vi "MB_TCP_7018.vi"(5 "Status Reference":T1, 6 "N":i32, 7 "Data Reference":T2, 9 "timeouts":T3={"conn_timeout"=1000, "reconn_timeout"=3000, "N attempt max"=3, "t_reset_TTL"=120000, "write_timeout"=10, "read_timeout"=500, "period"=100} {"t_reset_TTL" min=10 max=240000 step=1; "period" min=10 max=100000 step=1; "read_timeout" min=10 max=60000 step=1; "write_timeout" min=1 max=60000 step=1; "N attempt max" min=1 max=5 step=1; "reconn_timeout" min=10 max=240000 step=1; "conn_timeout" min=10 max=240000}, 10 "write enable":bool=TRUE, 11 "stop":bool) -> (0 "error out":errorcluster, 2 "errors":i32, 3 "Z3":u32)   [LabVIEW 2019, in "MB_TCP1.lvlib"]
uses:
  MB_TCP1.lvlib
  Timer Delay/Timers.lvlib
  NI_modbus_upd/NI_modbus_upd.lvlib
  NI_modbus_upd/MB Modbus Command.ctl
  ICPCON Registers/ICPCON Registers.lvlib
  ICPCON Status/ICPCON Status.lvlib
  Timer Delay/unix time 1ms.vi
  NI_modbus_upd/TCP/TCP.lvclass
  ICPCON Registers/Ctl/ICPCON Data.ctl
  ICPCON Status/Ctl/ICPCON Status.ctl
panel:
  out "stopped":bool
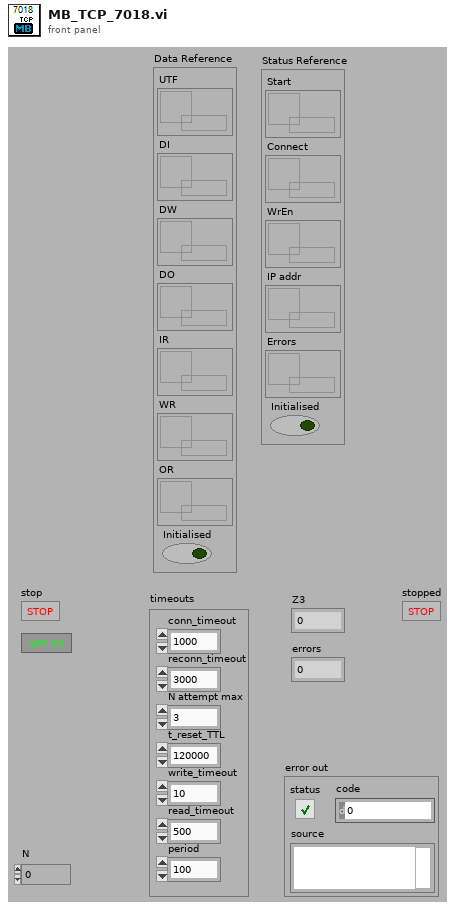
[diagram p1: front panel]
types:
  T1 = typedef "ICPCON Status.lvlib/ICPCON Status.ctl" = cluster{"Start":refnum<data-value>, "Connect":refnum<data-value>, "WrEn":refnum<data-value>, "IP addr":refnum<data-value>, "Errors":refnum<data-value>, "Initialised":bool}
  T2 = typedef "ICPCON Registers.lvlib/ICPCON Data.ctl" = cluster{"UTF":refnum<data-value>, "DI":refnum<data-value>, "DW":refnum<data-value>, "DO":refnum<data-value>, "IR":refnum<data-value>, "WR":refnum<data-value>, "OR":refnum<data-value>, "Initialised":bool}
  T3 = cluster{"conn_timeout":i32, "reconn_timeout":i32, "N attempt max":i32, "t_reset_TTL":i32, "write_timeout":i32, "read_timeout":i32, "period":i32}
  T4 = cluster{"Transaction ID":u16, "Protocol ID":u16, "Length":u16, "Unit ID":u8}
  T5 = typedef "NI_modbus_upd.lvlib/MB Modbus Command.ctl" = cluster{"Function Code":u8, "Starting Address":u16, "Quantity":u16, "Data":u16[], "Discrete":bool[]}
  T6 = cluster{"Remote IP Address":string, "Remote Port":u16}
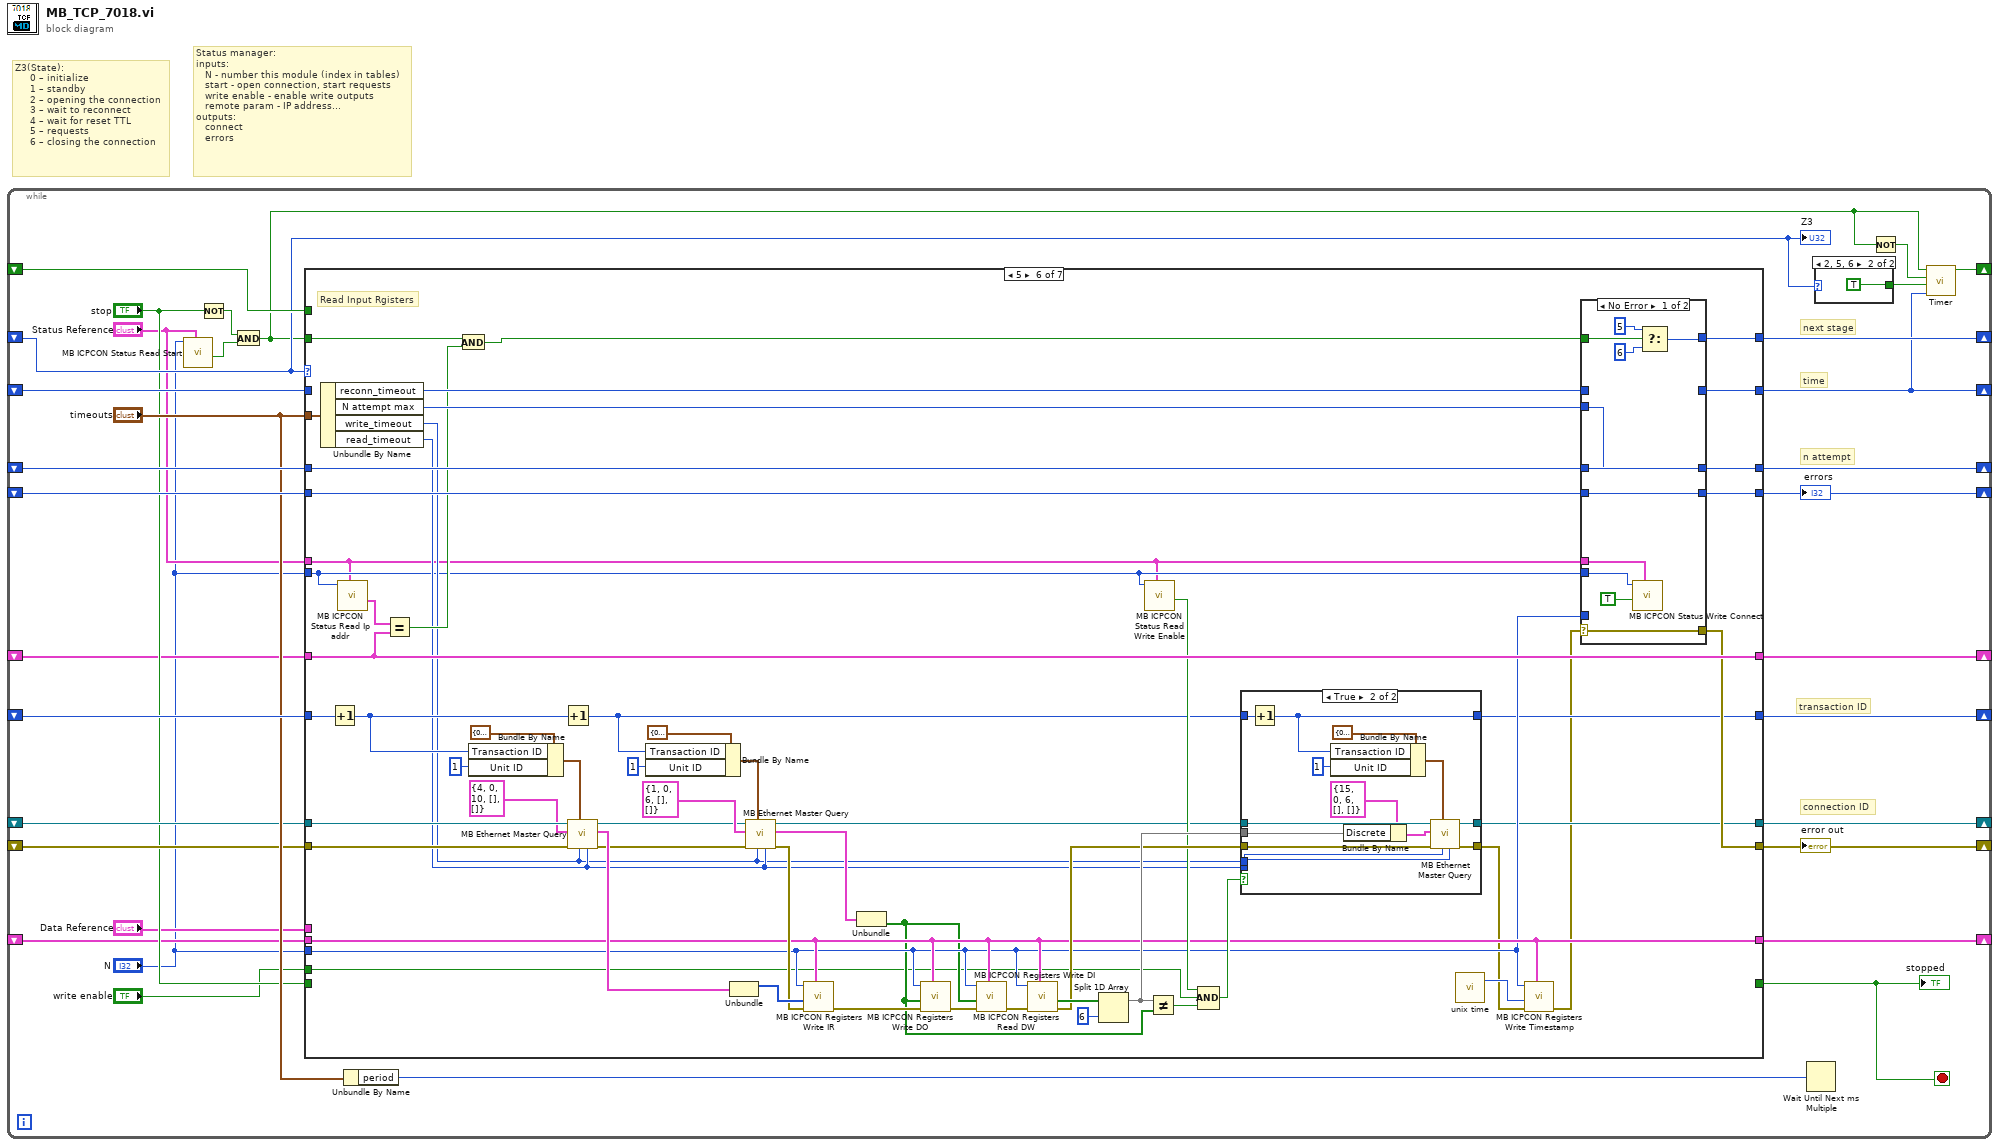
[diagram p0: block diagram]
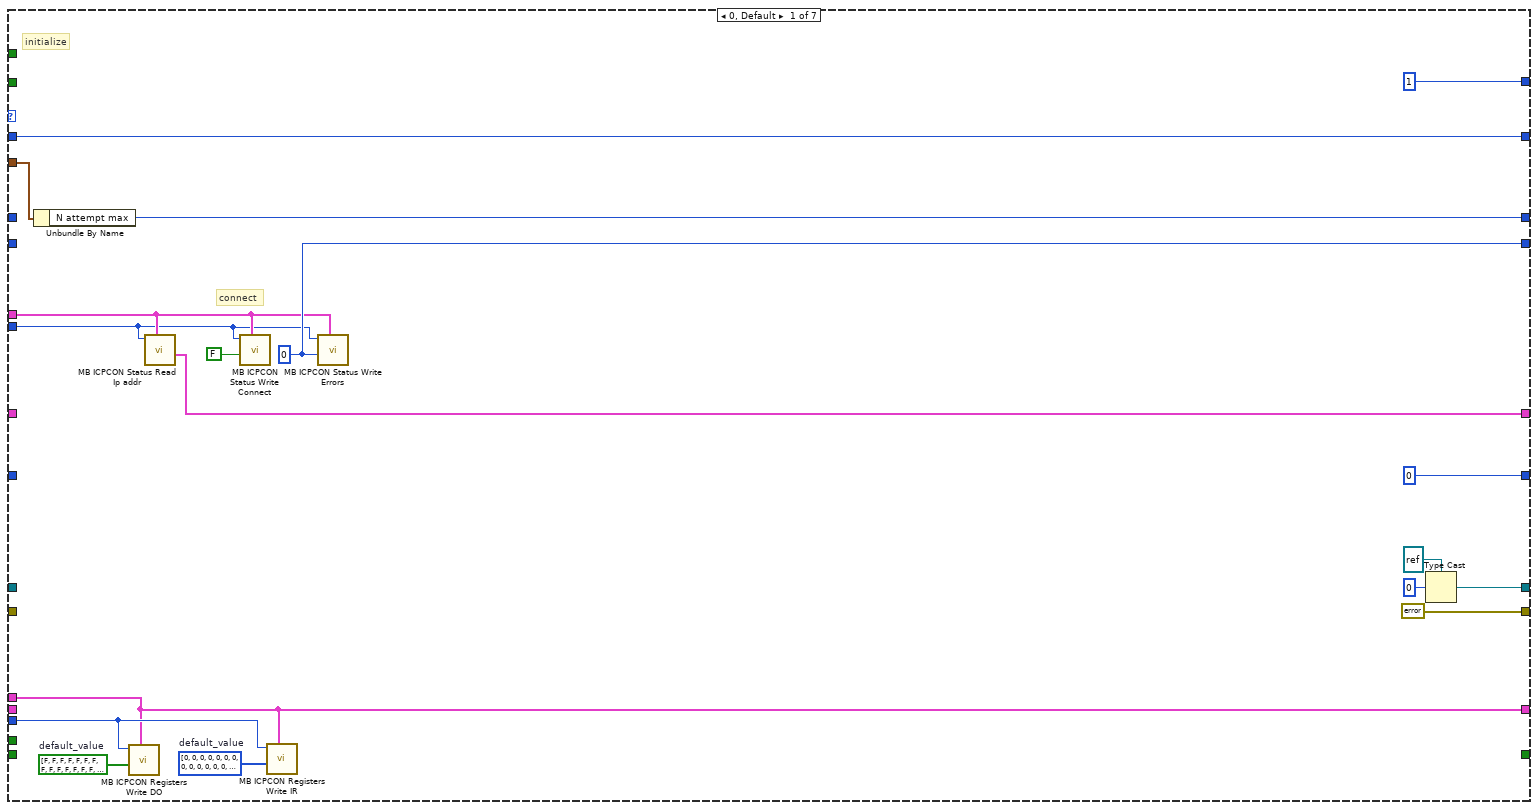
[diagram p2: hidden frame]
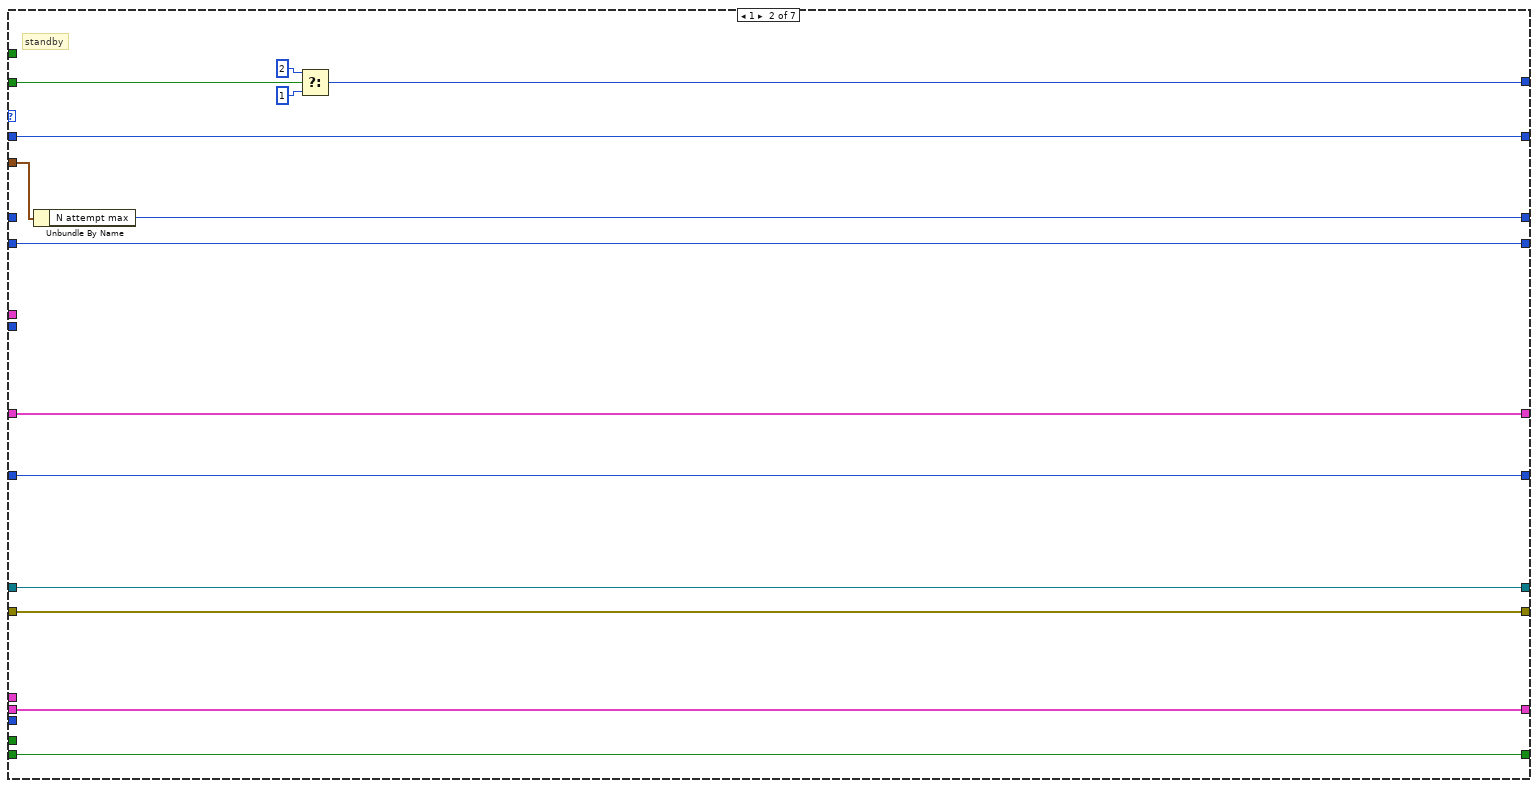
[diagram p3: hidden frame]
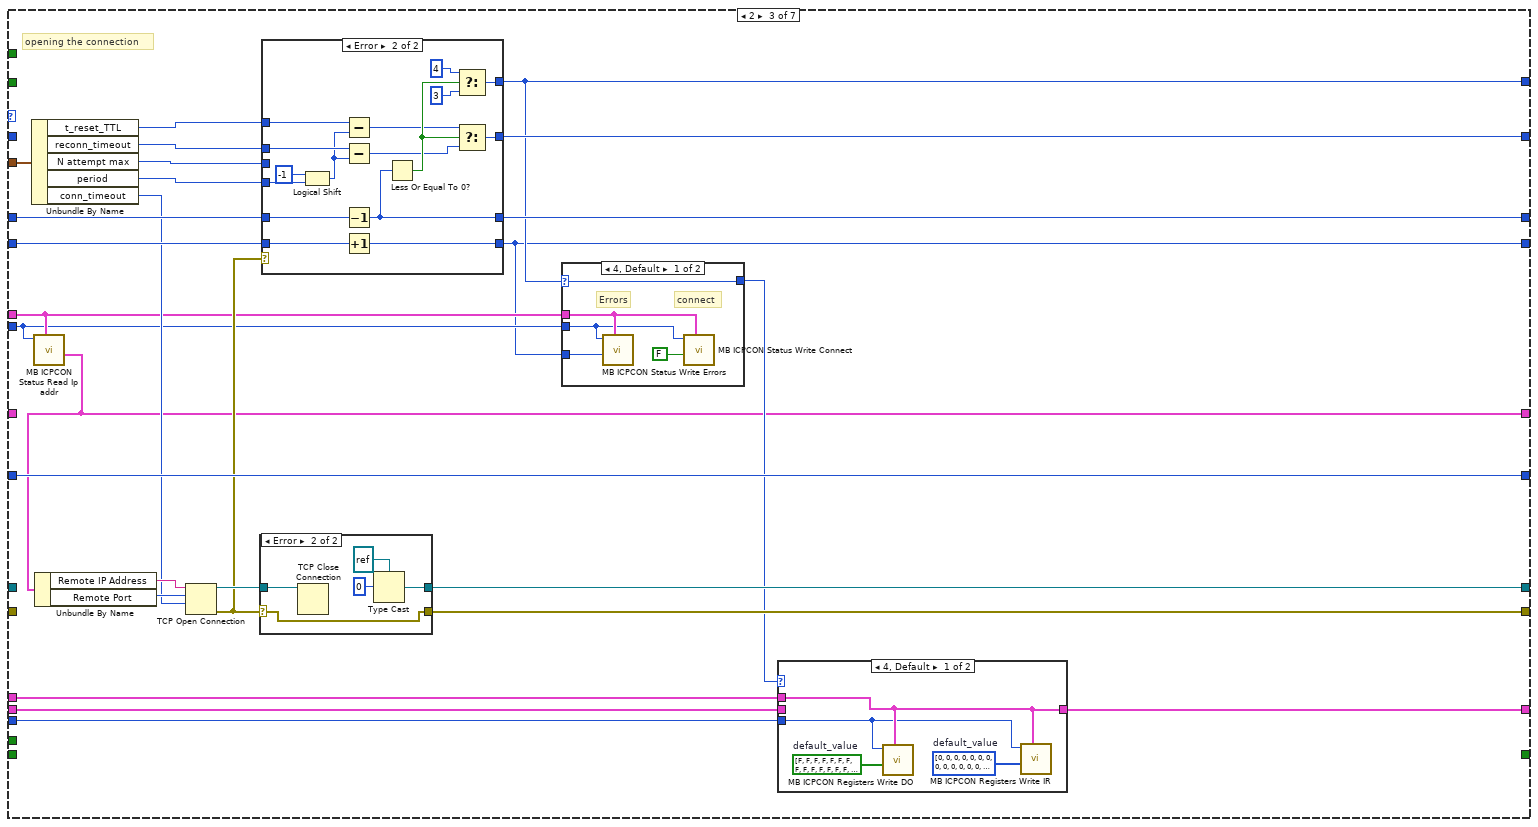
[diagram p4: hidden frame]
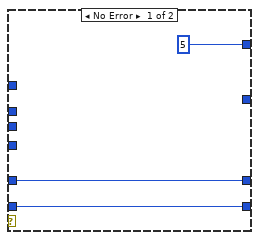
[diagram p8: hidden frame]
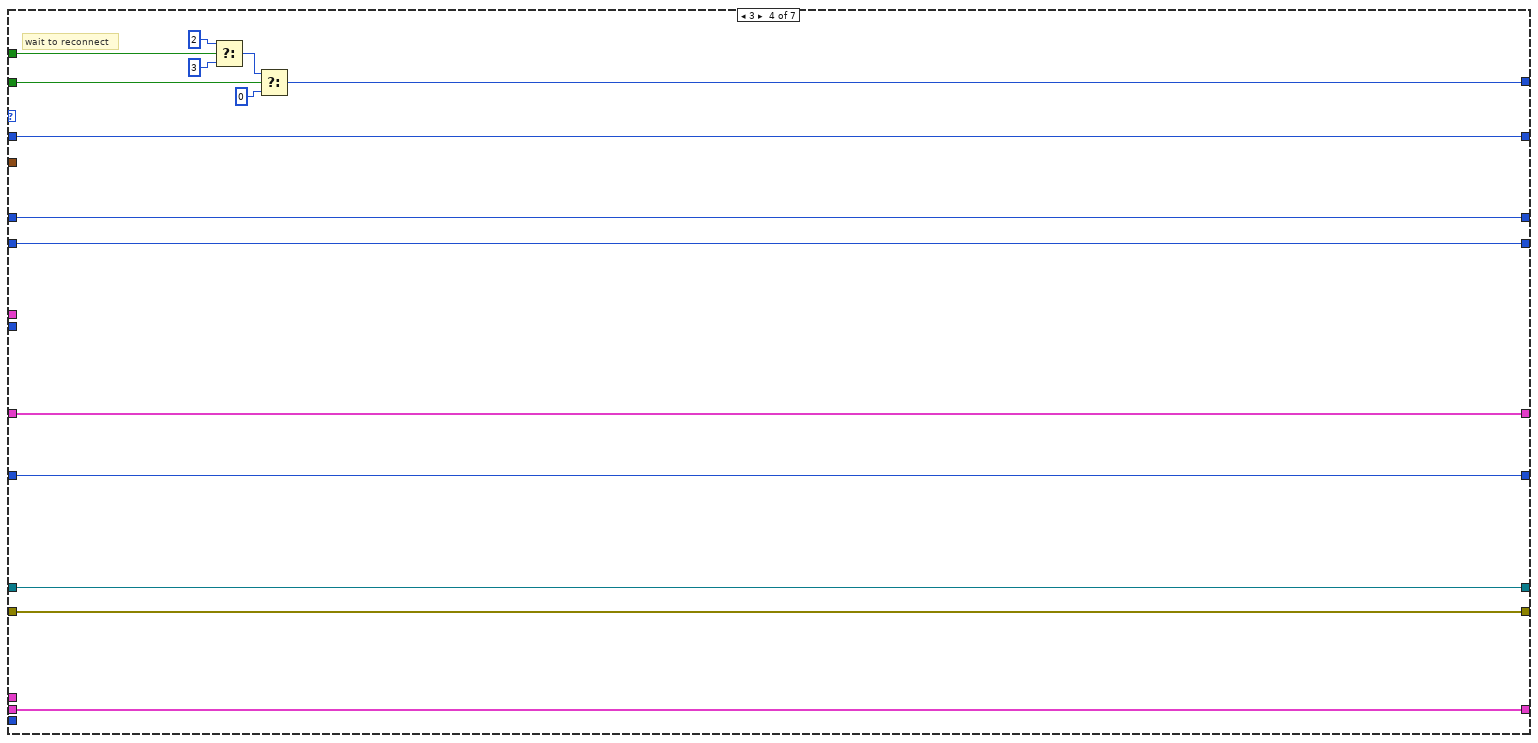
[diagram p9: hidden frame]
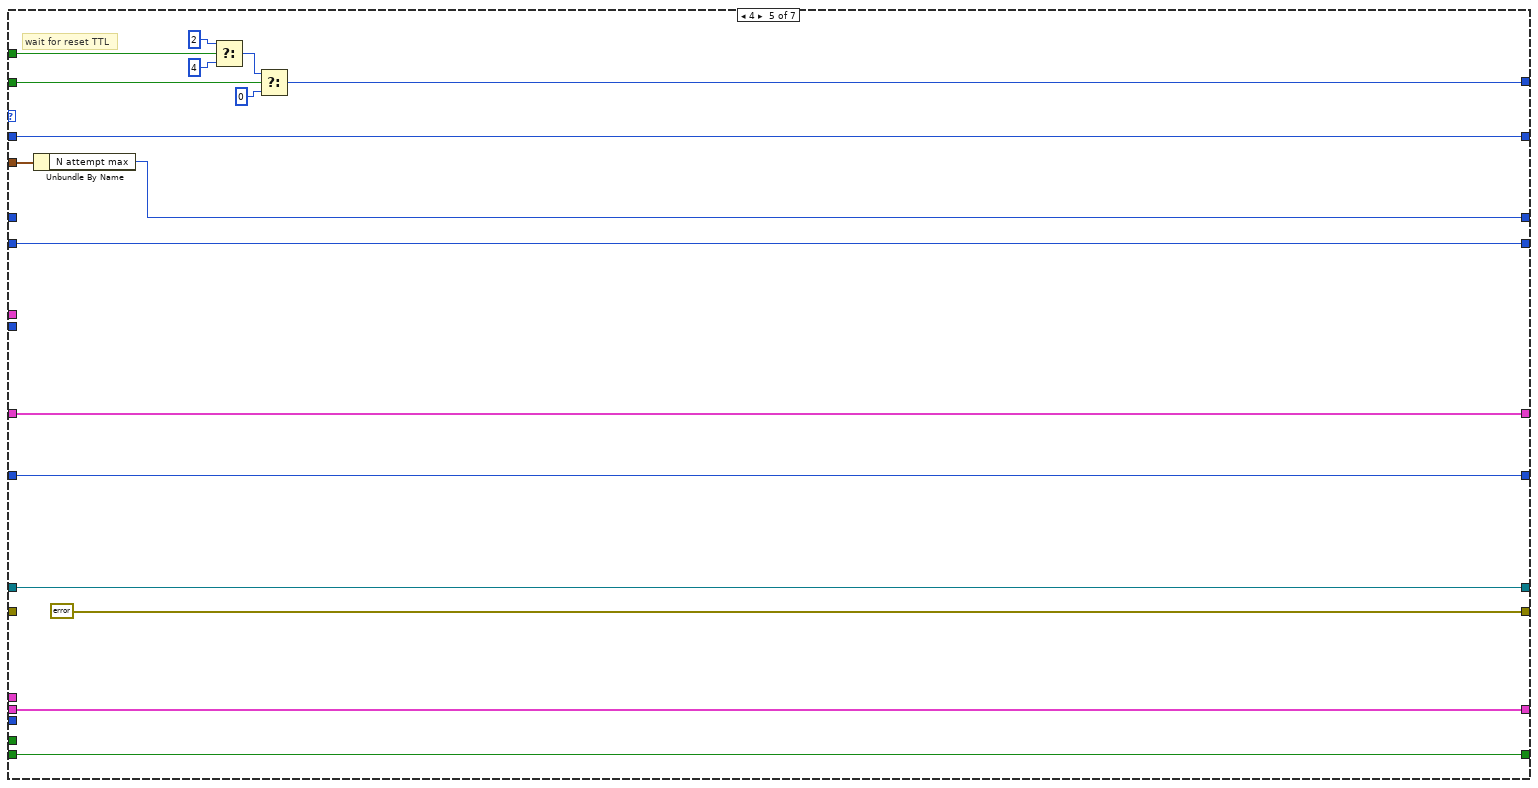
[diagram p10: hidden frame]
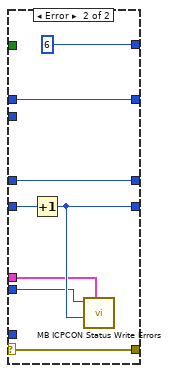
[diagram p12: hidden frame]
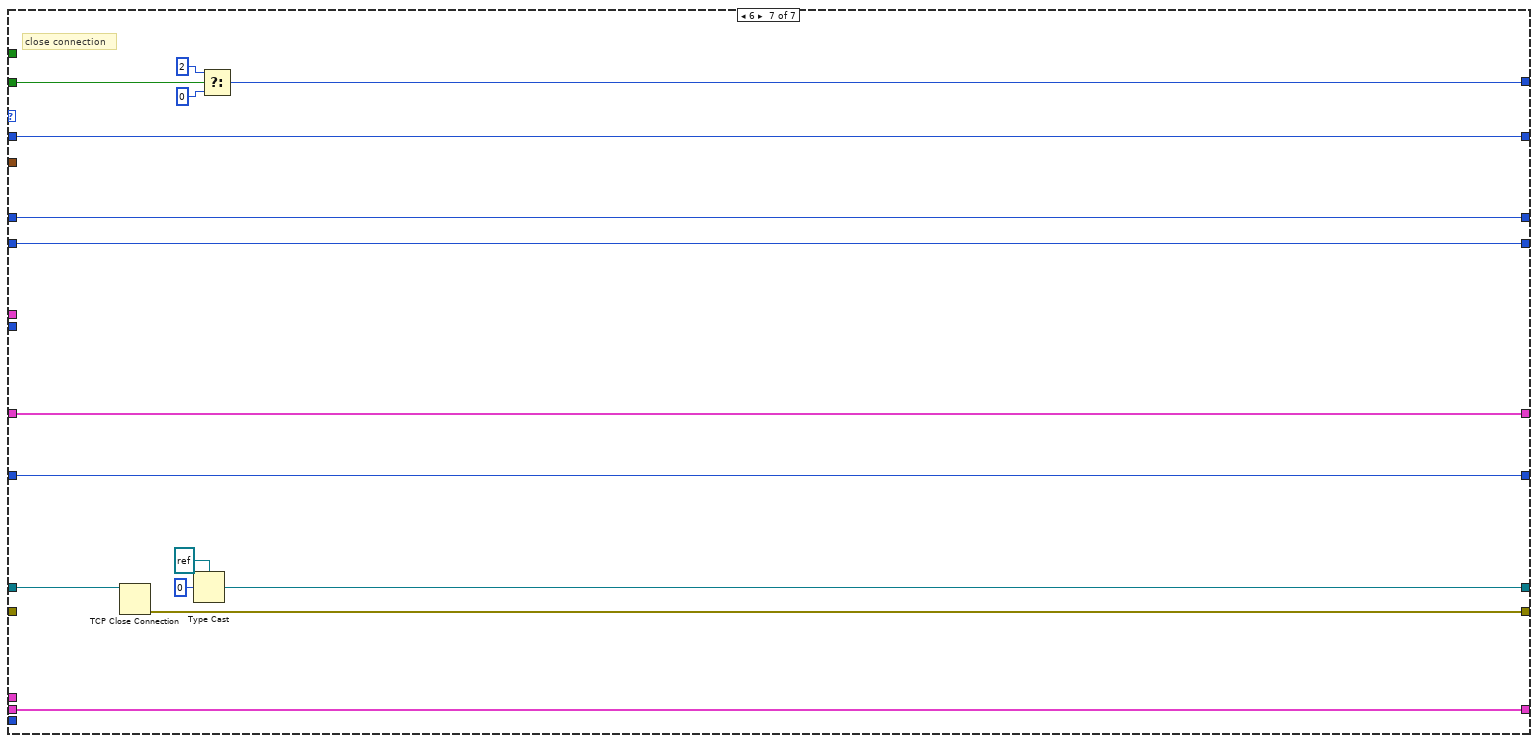
[diagram p13: hidden frame]
diagram:
  # "Status manager:\ninputs:\n   N - number this module (index in tables)\n   start - open connection, start requests\n   write enable - enable write outputs\n   remote param - IP address...\noutputs:\n   connect\n   errors"
  # "Z3(State):\n     0 – initialize \n     1 – standby\n     2 – opening the connection\n     3 – wait to reconnect\n     4 – wait for reset TTL\n     5 – requests\n     6 – closing the connection"
  n1 = while {
    shift-right: [w18] -> _
    shift-left: _ -> [w14]
    shift-right: [w17] -> _
    shift-left: _ -> [w32]
    shift-right: [w31] -> _
    shift-left: _ -> [w29]
    shift-right: [w30] -> _
    shift-left: _ -> [w28]
    shift-right: [w27] -> _
    shift-left: _ -> [w19]
    shift-right: [w26] -> _
    shift-left: _ -> [w20]
    shift-right: [w25] -> _
    shift-left: _ -> [w24]
    shift-right: [w16] -> _
    shift-left: _ -> [w15]
    shift-right: [w10] -> _
    shift-left: _ -> [w9]
    shift-right: [w7] -> _
    shift-left: _ -> [w6]
    stop <- w1 stop-if-true
    # "connection ID"
    # "transaction ID"
    # "n attempt"
    # "time"
    # "next stage"
    n2 = call "MB ICPCON Status Read Start.vi"("Status Reference"="Status Reference", "N"="N") -> ("Start"=w4:bool)  [unwired: 8 in, 1 out]
    n3 = Not(x="stop") -> (.not. x?=w12:bool)
    n4 = And(x=w12, y=w4) -> (x .and. y?=w13:bool)
    n5 = case shown="5" w14 {
      tunnel: [w49 w57 w78 w142 w147 w169 w265] -> w27
      tunnel: [errorcluster {"status"=FALSE, "code"=0, "source"=""} ("error out") w56 w76 w141 errorcluster {"status"=FALSE, "code"=0, "source"=""} ("error out") w186 w266] -> w26
      tunnel: w19 -> [_ w57 _ w142 w147 w208 w262]
      tunnel: w20 -> [_ w56 _ w141 _ w207 _]
      tunnel: w24 -> [_ w65 w92 w144 w161 w217 w267]
      tunnel: [u16 0 ("x") w65 w92 w144 w161 w171 w267] -> w25
      tunnel: [w44 w61 w88 w143 w157 w215 w259] -> w31
      tunnel: w29 -> [_ _ w89 w143 _ w215 w259]
      tunnel: [w36 w64 w66 w140 w160 w214 w264] -> w30
      tunnel: w28 -> [_ w64 w91 w140 w160 w213 w264]
      tunnel: [w46 w63 w85 w139 w159 w210 w263] -> w17
      tunnel: w32 -> [w46 w63 _ w139 w159 _ w263]
      tunnel: "timeouts" -> [w45 w62 w90 _ w158 w216 _]
      tunnel: w13 -> [_ w55 _ w135 w149 w202 w260]
      tunnel: [u32 1 w58 w75 w132 w152 w209 w255] -> w18
      tunnel: w15 -> [_ _ _ w133 w151 _ _]
      tunnel: "N" -> [w40 _ w72 _ _ w174 _]
      tunnel: "stop" -> [_ w54 _ _ w148 _ _]
      tunnel: [_ w54 _ _ w148 _ _] -> w1
      tunnel: [w37 w53 w69 w131 w146 w200 w254] -> w10
      tunnel: w9 -> [_ w53 _ w131 w146 w200 w254]
      tunnel: "Data Reference" -> [w39 _ w71 _ _ _ _]
      tunnel: [w39 w52 w74 w130 w145 w175 w253] -> w7
      tunnel: w6 -> [_ w52 w70 w130 w145 w175 w253]
      tunnel: "write enable" -> [_ _ _ _ _ w164 _]
      tunnel: "Status Reference" -> [w35 _ w68 _ _ w165 _]
      tunnel: "N" -> [w34 _ w67 _ _ w166 _]
      frame 0, Default {
        w36 = 0 ("N attempt max")
        w41 = bool[] [FALSE, FALSE, FALSE, FALSE, FALSE, FALSE, FALSE, FALSE, FALSE, FALSE, FALSE, FALSE, FALSE, FALSE, FALSE, FALSE, FALSE, FALSE, FALSE, FALSE, FALSE, FALSE, FALSE, FALSE, FALSE, FALSE, FALSE, FALSE, FALSE, FALSE, FALSE, FALSE]  # default_value
        w42 = u16[] [0, 0, 0, 0, 0, 0, 0, 0, 0, 0, 0, 0, 0, 0, 0, 0, 0, 0, 0, 0]  # default_value
        # "connect"
        # "initialize"
        n6 = Unbundle By Name(w45) -> ("N attempt max"=w44:i32)
        n7 = call "MB ICPCON Registers Write DO.vi"("Data Reference"=w39, "Bits In"=w41, "N"=w40) -> ()  [unwired: 8 in, 1 out]
        n8 = call "MB ICPCON Status Read Ip addr.vi"("Status Reference"=w35, "N"=w34) -> ("IP address"=w37:T6)  [unwired: 8 in, 1 out]
        n9 = call "MB ICPCON Status Write Connect.vi"("Status Reference"=w35, "Connect"=FALSE ("connect"), "N"=w34) -> ()  [unwired: 8 in, 1 out]
        n10 = call "MB ICPCON Registers Write IR.vi"("Data Reference"=w39, "Words In"=w42, "N"=w40) -> ()  [unwired: 8 in, 1 out]
        n11 = call "MB ICPCON Status Write Errors.vi"("Status Reference"=w35, "Errors"=w36, "N"=w34) -> ()  [unwired: 8 in, 1 out]
        n12 = Type Cast(type=refnum<k5> refnum ("connection ID"), x=u32 0) -> (*(type *) &x=w49:refnum<k5>)
      }
      frame 1 {
        # "standby"
        n13 = Unbundle By Name(w62) -> ("N attempt max"=w61:i32)
        n14 = Select(t=u32 2, s=w55, f=u32 1) -> (s? t:f=w58:u32)
      }
      frame 2 {
        # "opening the connection"
        n15 = Unbundle By Name(w90) -> ("t_reset_TTL"=w84:i32, "reconn_timeout"=w86:i32, "N attempt max"=w87:i32, "period"=w81:i32, "conn_timeout"=w80:i32)
        n16 = call "MB ICPCON Status Read Ip addr.vi"("Status Reference"=w68, "N"=w67) -> ("IP address"=w69:T6)  [unwired: 8 in, 1 out]
        n17 = Unbundle By Name(w69) -> ("Remote IP Address"=w83:string, "Remote Port"=w82:u16)
        n18 = TCP Open Connection(address=w83, remote port or service name=w82, timeout ms (60000)=w80) -> (connection ID=w79:refnum<k5>, error out=w77:errorcluster)  [unwired: 2 in]
        n19 = case shown="Error" w77 {
          selector: w77 -> [w104 w106]
          tunnel: w79 -> [w105 w109]
          tunnel: [w105 w108] -> w78
          tunnel: [w104 w106] -> w76
          frame No Error {
          }
          frame Error {
            n20 = TCP Close Connection(connection ID=w109) -> ()  [unwired: 2 in, 2 out]
            n21 = Type Cast(type=refnum<k5> refnum ("connection ID"), x=u32 0) -> (*(type *) &x=w108:refnum<k5>)
          }
        }
        n22 = case shown="Error" w77 {
          tunnel: w91 -> [w113 w129]
          tunnel: [w113 w128] -> w66
          tunnel: w89 -> [w112 w127]
          tunnel: [w112 w126] -> w88
          tunnel: w87 -> [_ _]
          tunnel: [u32 5 w123] -> w75
          tunnel: w86 -> [_ w122]
          tunnel: [_ w121] -> w85
          tunnel: w84 -> [_ w118]
          tunnel: w81 -> [_ w116]
          frame No Error {
          }
          frame Error {
            n23 = Logical Shift(y=i16 -1, x=w116) -> (x << y=w114:i32)
            n24 = Subtract(x=w118, y=w114) -> (x-y=w117:i32)
            n25 = Subtract(x=w122, y=w114) -> (x-y=w119:i32)
            n26 = Decrement(x=w127) -> (x-1=w126:i32)
            n27 = Increment(x=w129) -> (x+1=w128:i32)
            n28 = Less Or Equal To 0?(x=w126) -> (x <= 0?=w120:bool)
            n29 = Select(t=u32 4, s=w120, f=u32 3) -> (s? t:f=w123:u32)
            n30 = Select(t=w117, s=w120, f=w119) -> (s? t:f=w121:i32)
          }
        }
        n31 = case shown="4, Default" w75 {
          selector: w75 -> [w102 w103]
          tunnel: [w102 w103] -> w73
          tunnel: w68 -> [w100 _]
          tunnel: w67 -> [w99 _]
          tunnel: w66 -> [w98 _]
          frame 4, Default {
            # "Errors"
            # "connect"
            n32 = call "MB ICPCON Status Write Errors.vi"("Status Reference"=w100, "Errors"=w98, "N"=w99) -> ()  [unwired: 8 in, 1 out]
            n33 = call "MB ICPCON Status Write Connect.vi"("Status Reference"=w100, "Connect"=FALSE ("f"), "N"=w99) -> ()  [unwired: 8 in, 1 out]
          }
          frame 3, 5 {
          }
        }
        n34 = case shown="4, Default" w73 {
          tunnel: w72 -> [w93 _]
          tunnel: w70 -> [_ w97]
          tunnel: [w94 w97] -> w74
          tunnel: w71 -> [w94 _]
          frame 4, Default {
            w95 = bool[] [FALSE, FALSE, FALSE, FALSE, FALSE, FALSE, FALSE, FALSE, FALSE, FALSE, FALSE, FALSE, FALSE, FALSE, FALSE, FALSE, FALSE, FALSE, FALSE, FALSE, FALSE, FALSE, FALSE, FALSE, FALSE, FALSE, FALSE, FALSE, FALSE, FALSE, FALSE, FALSE]  # default_value
            w96 = u16[] [0, 0, 0, 0, 0, 0, 0, 0, 0, 0, 0, 0, 0, 0, 0, 0, 0, 0, 0, 0]  # default_value
            n35 = call "MB ICPCON Registers Write DO.vi"("Data Reference"=w94, "Bits In"=w95, "N"=w93) -> ()  [unwired: 8 in, 1 out]
            n36 = call "MB ICPCON Registers Write IR.vi"("Data Reference"=w94, "Words In"=w96, "N"=w93) -> ()  [unwired: 8 in, 1 out]
          }
          frame 3, 5 {
          }
        }
      }
      frame 3 {
        # "wait to reconnect"
        n37 = Select(t=u32 2, s=w133, f=u32 3) -> (s? t:f=w134:u32)
        n38 = Select(t=w134, s=w135, f=u32 0) -> (s? t:f=w132:u32)
      }
      frame 4 {
        # "wait for reset TTL"
        n39 = Unbundle By Name(w158) -> ("N attempt max"=w157:i32)
        n40 = Select(t=u32 2, s=w151, f=u32 4) -> (s? t:f=w153:u32)
        n41 = Select(t=w153, s=w149, f=u32 0) -> (s? t:f=w152:u32)
      }
      frame 5 {
        # "Read Input Rgisters"
        n42 = Unbundle By Name(w216) -> ("reconn_timeout"=w211:i32, "N attempt max"=w212:i32, "write_timeout"=w172:i32, "read_timeout"=w173:i32)
        n43 = Increment(x=w217) -> (x+1=w194:u16)
        n44 = call "MB ICPCON Status Read Ip addr.vi"("Status Reference"=w165, "N"=w166) -> ("IP address"=w184:T6)  [unwired: 8 in, 1 out]
        n45 = Equal?(x=w184, y=w200) -> (x = y?=w199:bool)
        n46 = And(x=w202, y=w199) -> (x .and. y?=w201:bool)
        n47 = Bundle By Name(cluster=T4 {"Transaction ID"=0, "Protocol ID"=0, "Length"=0, "Unit ID"=0} ("MBAP Header"), "Transaction ID"=w194, "Unit ID"=u8 1) -> (w203:T4)
        n48 = Increment(x=w194) -> (x+1=w171:u16)
        n49 = call "MB Ethernet Master Query.vi"(4:w173, 6:w172, "MBAP Header"=w203, "error in (no error)"=w207, "Modbus Command"=T5 {"Function Code"=4, "Starting Address"=0, "Quantity"=10, "Data"=[], "Discrete"=[]}, "TCP in"=w208) -> ("error out"=w192:errorcluster, "Registers"=w206:cluster{"Registers":u16[], "Discrete":bool[]}, "TCP out"=w190:refnum<class "TCP.lvclass">)  [unwired: 2 in, 1 out]
        n50 = Bundle By Name(cluster=T4 {"Transaction ID"=0, "Protocol ID"=0, "Length"=0, "Unit ID"=0} ("MBAP Header"), "Transaction ID"=w171, "Unit ID"=u8 1) -> (w197:T4)
        n51 = Unbundle(w206) -> ("Registers"=w188:u16[])  [unwired: 1 out]
        n52 = call "MB Ethernet Master Query.vi"(4:w173, 6:w172, "MBAP Header"=w197, "error in (no error)"=w192, "Modbus Command"=T5 {"Function Code"=1, "Starting Address"=0, "Quantity"=6, "Data"=[], "Discrete"=[]} ("MODBUS Command"), "TCP in"=w190) -> ("error out"=w187:errorcluster, "Registers"=w191:cluster{"Registers":u16[], "Discrete":bool[]}, "TCP out"=w170:refnum<class "TCP.lvclass">)  [unwired: 2 in, 1 out]
        n53 = call "MB ICPCON Registers Write IR.vi"("Data Reference"=w175, "error in (no error)"=w187, "Words In"=w188, "N"=w174) -> ("error out"=w189:errorcluster)  [unwired: 7 in]
        n54 = Unbundle(w191) -> ("Discrete"=w167:bool[])  [unwired: 1 out]
        n55 = call "MB ICPCON Registers Write DO.vi"("Data Reference"=w175, "error in (no error)"=w189, "Bits In"=w167, "N"=w174) -> ("error out"=w183:errorcluster)  [unwired: 7 in]
        n56 = call "MB ICPCON Registers Write DI.vi"("Data Reference"=w175, "error in (no error)"=w183, "Bits In"=w167, "N"=w174) -> ("error out"=w168:errorcluster)  [unwired: 7 in]
        n57 = call "MB ICPCON Registers Read DW.vi"("Data Reference"=w175, "error in (no error)"=w168, "N"=w174) -> ("error out"=w177:errorcluster, "Bits out"=w180:bool[])  [unwired: 7 in]
        n58 = Split 1D Array(array=w180, index=6 ("length")) -> (first subarray=w178:bool[])  [unwired: 1 out]
        n59 = call "MB ICPCON Status Read Write Enable.vi"("Status Reference"=w165, "N"=w166) -> ("Write Enable"=w176:bool)  [unwired: 8 in, 1 out]
        n60 = Not Equal?(x=w178, y=w167) -> (x != y?=w182:bool)
        n61 = Compound Arithmetic op=AND(w176, w164, w182) -> (w181:bool)
        n62 = case shown="True" w181 {
          tunnel: w173 -> [_ w232]
          tunnel: w172 -> [_ w231]
          tunnel: w171 -> [w219 w230]
          tunnel: [w219 w229] -> _
          tunnel: w177 -> [w218 w227]
          tunnel: [w218 w226] -> w163
          tunnel: w170 -> [w220 w225]
          tunnel: [w220 w224] -> w169
          tunnel: w178 -> [_ w221]
          frame False {
          }
          frame True {
            n63 = Increment(x=w230) -> (x+1=w229:u16)
            n64 = Bundle By Name(cluster=T4 {"Transaction ID"=0, "Protocol ID"=0, "Length"=0, "Unit ID"=0} ("MBAP Header"), "Transaction ID"=w229, "Unit ID"=u8 1) -> (w233:T4)
            n65 = Bundle By Name(cluster=T5 {"Function Code"=15, "Starting Address"=0, "Quantity"=6, "Data"=[], "Discrete"=[]} ("MODBUS Command"), "Discrete"=w221) -> (w222:T5)
            n66 = call "MB Ethernet Master Query.vi"(4:w232, 6:w231, "MBAP Header"=w233, "error in (no error)"=w227, "Modbus Command"=w222, "TCP in"=w225) -> ("error out"=w226:errorcluster, "TCP out"=w224:refnum<class "TCP.lvclass">)  [unwired: 2 in, 2 out]
          }
        }
        n67 = call-poly "unix time.vi"() -> ("unix time (ms)"=w185:u64)  [unwired: 2 in, 1 out]
        n68 = call "MB ICPCON Registers Write Timestamp.vi"("Data Reference"=w175, "error in (no error)"=w163, "UTF"=w185, "N"=w174) -> ("error out"=w162:errorcluster)  [unwired: 7 in]
        n69 = case shown="No Error" w162 {
          selector: w162 -> [w238 w248]
          tunnel: w213 -> [w239 w252]
          tunnel: [w239 w247] -> w214
          tunnel: [w241 u32 6] -> w209
          tunnel: w215 -> [_ w250]
          tunnel: w212 -> [w244 _]
          tunnel: [w244 w250] -> _
          tunnel: w211 -> [_ w249]
          tunnel: [_ w249] -> w210
          tunnel: w201 -> [w240 _]
          tunnel: w174 -> [_ _]
          tunnel: [w238 w248] -> w186
          tunnel: w165 -> [w236 w246]
          tunnel: w166 -> [w235 w245]
          frame No Error {
            n70 = call "MB ICPCON Status Write Connect.vi"("Status Reference"=w236, "Connect"=TRUE ("f"), "N"=w235) -> ()  [unwired: 8 in, 1 out]
            n71 = Select(t=u32 5, s=w240, f=u32 6) -> (s? t:f=w241:u32)
          }
          frame Error {
            n72 = Increment(x=w252) -> (x+1=w247:i32)
            n73 = call "MB ICPCON Status Write Errors.vi"("Status Reference"=w246, "Errors"=w247, "N"=w245) -> ()  [unwired: 8 in, 1 out]
          }
        }
      }
      frame 6 {
        # "close connection"
        n74 = TCP Close Connection(connection ID=w262) -> (error out=w266:errorcluster)  [unwired: 2 in, 1 out]
        n75 = Type Cast(type=refnum<k5> refnum ("connection ID"), x=u32 0) -> (*(type *) &x=w265:refnum<k5>)
        n76 = Select(t=u32 2, s=w260, f=u32 0) -> (s? t:f=w255:u32)
      }
    }
    "error out" <- w26
    "errors" <- w30
    "stopped" <- w1
    n77 = Unbundle By Name("timeouts") -> ("period"=w22:i32)
    n78 = Wait Until Next ms Multiple(millisecond multiple=w22) -> ()  [unwired: 1 out]
    n79 = case shown="2, 5, 6" w14 {
      tunnel: [_ TRUE] -> w21
      frame 0, Default {
      }
      frame 2, 5, 6 {
      }
    }
    n80 = Not(x=w13) -> (.not. x?=w33:bool)
    n81 = call "Timer.vi"("ms"=w17, "Load (F)"=w21, "Reset (F)"=w33, "Start (T)"=w13) -> ("End"=w16:bool)  [unwired: 5 in, 1 out]
    "Z3" <- w14
  }
